vi "CASE STRUCTURE WITH ENUM.vi"(5 "Enum":enum16{"RED", "YELLOW", "GREEN"}(ring)) -> (0 "GREEN":bool, 1 "YELLOW":bool, 2 "RED":bool)   [LabVIEW 2018]
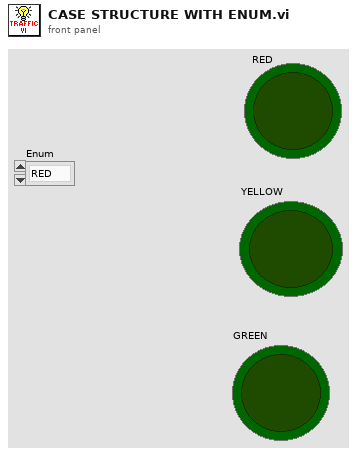
[diagram p1: front panel]
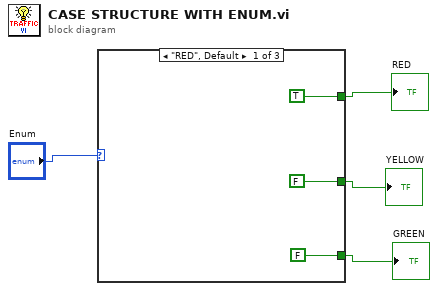
[diagram p0: block diagram]
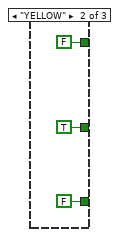
[diagram p2: hidden frame]
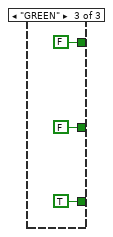
[diagram p3: hidden frame]
diagram:
  n1 = case shown="\"RED\", Default" "Enum" {
    tunnel: [TRUE FALSE FALSE] -> w4
    tunnel: [FALSE TRUE FALSE] -> w3
    tunnel: [FALSE FALSE TRUE] -> w2
    frame "RED", Default {
    }
    frame "YELLOW" {
    }
    frame "GREEN" {
    }
  }
  "RED" <- w4
  "YELLOW" <- w3
  "GREEN" <- w2
